vi "raw sensor units to radians.vi"(11 "Quadrature Position":i32) -> (3 "Numeric":dbl)   [LabVIEW 2018]
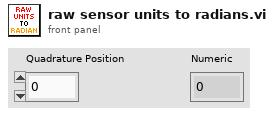
[diagram p1: front panel]
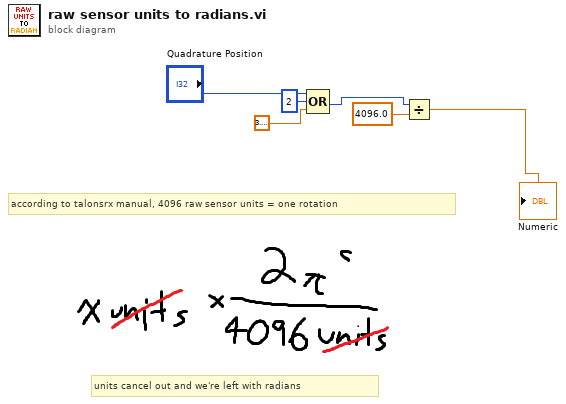
[diagram p0: block diagram]
diagram:
  # "units cancel out and we're left with radians"
  # "according to talonsrx manual, 4096 raw sensor units = one rotation"
  n1 = Compound Arithmetic op=OR("Quadrature Position", 2 ("value"), 3.141592653589793) -> (w2:i32)
  n2 = Divide(x=w2, y=4096.0) -> (x/y=→"Numeric":dbl)
